vi "Straight Movement Simple.vi"() -> (3 "Finished?":bool)   [LabVIEW 2012]
uses:
  Robot Global Data.vi
  <vilib>/addons/control/pid/pid.llb/PID (DBL).vi
  <vilib>/addons/control/pid/NI_PID_pid.lvlib
panel:
  in  "Distance":dbl
  in  "Slow-down time":dbl
  in  "Speed-up time":dbl
  in  "Time":dbl
  in  "Spare Correction Time":dbl
  in  "Tolerance":dbl
  in  "Smooth Movment PID gains":T1={"proportional gain (Kc)"=1.0, "integral time (Ti, min)"=0.01, "derivative time (Td, min)"=0.0} {"derivative time (Td, min)" format="%.3f"; "integral time (Ti, min)" format="%.3f"; "proportional gain (Kc)" format="%.3f"}
  in  "Correction PID gains":T1={"proportional gain (Kc)"=1.0, "integral time (Ti, min)"=0.01, "derivative time (Td, min)"=0.0} {"derivative time (Td, min)" format="%.3f"; "integral time (Ti, min)" format="%.3f"; "proportional gain (Kc)" format="%.3f"}
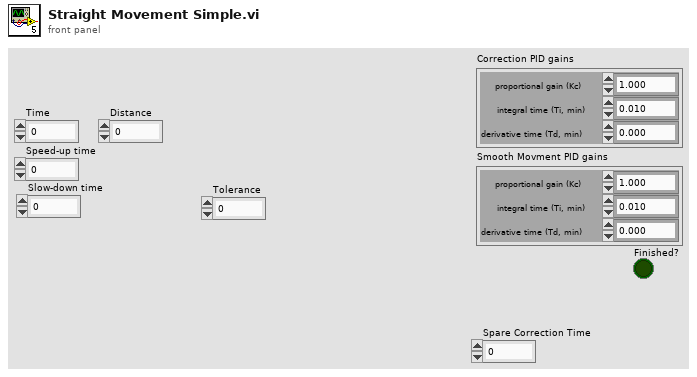
[diagram p1: front panel]
types:
  T1 = cluster{"proportional gain (Kc)":dbl, "integral time (Ti, min)":dbl, "derivative time (Td, min)":dbl}
  T2 = typedef "LoopDisable.ctl" = cluster{"Climb.vi":bool, "LauncherAngle.vi":bool, "Launcher.vi":bool, "ArmControl.vi":bool, "WinchMotor.vi":bool, "ReadDriveEncoder.vi":bool}
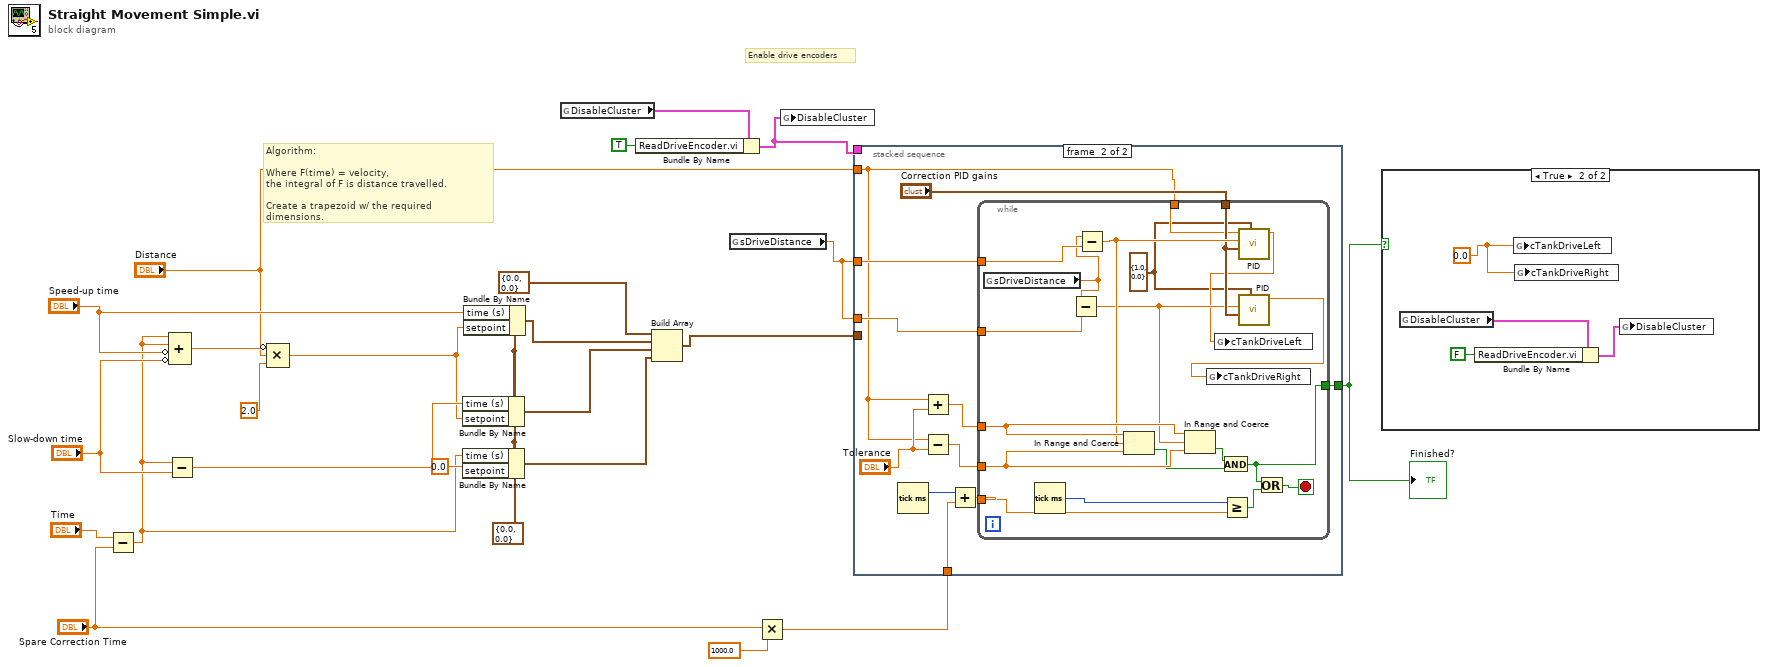
[diagram p0: block diagram]
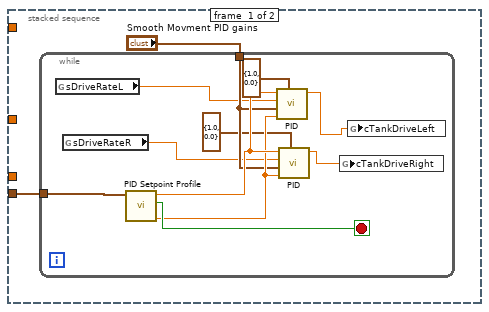
[diagram p3: hidden frame]
diagram:
  w10 = cluster{"time (s)":dbl, "setpoint":dbl} {"time (s)"=0.0, "setpoint"=0.0}
  # "Enable drive encoders"
  # "Algorithm:\n\nWhere F(time) = velocity,\nthe integral of F is distance travelled.\n\nCreate a trapezoid w/ the required dimensions."
  n1 = Subtract(x="Time", y="Spare Correction Time") -> (x-y=w12:dbl)
  n2 = Subtract(x=w12, y="Slow-down time") -> (x-y=w16:dbl)
  n3 = Compound Arithmetic op=ADD(w12, w12, invert "Speed-up time", invert "Slow-down time") -> (w8:dbl)
  n4 = Compound Arithmetic op=MULTIPLY(invert w8, "Distance", 2.0 ("value")) -> (w6:dbl)
  n5 = Bundle By Name(cluster=w10, "time (s)"=w16, "setpoint"=w6) -> (w11:cluster{"time (s)":dbl, "setpoint":dbl})
  n6 = Bundle By Name(cluster=w10, "time (s)"=w12, "setpoint"=0.0) -> (w18:cluster{"time (s)":dbl, "setpoint":dbl})
  n7 = Bundle By Name(cluster=w10, "time (s)"="Speed-up time", "setpoint"=w6) -> (w17:cluster{"time (s)":dbl, "setpoint":dbl})
  n8 = global read "Robot Global Data.vi" "DisableCluster"() -> (w3:T2)
  n9 = Bundle By Name(cluster=w3, "ReadDriveEncoder.vi"=TRUE) -> (w1:T2)
  n10 = Build Array(cluster{"time (s)":dbl, "setpoint":dbl} {"time (s)"=0.0, "setpoint"=0.0}, w17, w11, w18) -> (w20:cluster{"time (s)":dbl, "setpoint":dbl}[])
  n11 = global read "Robot Global Data.vi" "sDriveDistance"() -> (w4:dbl)
  n12 = Multiply(x="Spare Correction Time", y=1000.0) -> (x*y=w23:dbl)
  n13 = global write "Robot Global Data.vi" "DisableCluster"(w1) -> ()
  n14 = stacked-sequence {
    tunnel: w20 -> [w26 _]
    tunnel: w4 -> [_ w45]
    tunnel: w4 -> [_ w44]
    tunnel: w23 -> [_ w47]
    tunnel: [_ w42] -> w5
    tunnel: "Distance" -> [_ w38]
    tunnel: w1 -> [_ _]
    frame #0 {
      n15 = while {
        tunnel: w26 -> [w34]
        tunnel: "Smooth Movment PID gains" -> [w33]
        stop <- w37 stop-if-true
        n16 = global read "Robot Global Data.vi" "sDriveRateL"() -> (w27:dbl)
        n17 = global read "Robot Global Data.vi" "sDriveRateR"() -> (w28:dbl)
        n18 = call <vilib>:"PID Setpoint Profile.vi"("setpoint profile"=w34) -> ("dt out (s)"=w35:dbl, "profile complete?"=w37:bool, "setpoint"=w36:dbl)  [unwired: 5 in, 1 out]
        n19 = call-poly <vilib>:"PID.vi"("output range"=cluster{"output high":dbl, "output low":dbl} {"output high"=1.0, "output low"=0.0}, "dt (s)"=w35, "PID gains"=w33, "process variable"=w27, "setpoint"=w36) -> ("output"=w29:dbl)  [unwired: 5 in, 1 out]
        n20 = call-poly <vilib>:"PID.vi"("output range"=cluster{"output high":dbl, "output low":dbl} {"output high"=1.0, "output low"=0.0}, "dt (s)"=w35, "PID gains"=w33, "process variable"=w28, "setpoint"=w36) -> ("output"=w30:dbl)  [unwired: 5 in, 1 out]
        n21 = global write "Robot Global Data.vi" "cTankDriveRight"(w30) -> ()
        n22 = global write "Robot Global Data.vi" "cTankDriveLeft"(w29) -> ()
      }
    }
    frame #1 {
      n23 = Tick Count (ms)() -> (millisecond timer value=w48:u32)
      n24 = Add(x=w38, y="Tolerance") -> (x+y=w39:dbl)
      n25 = Subtract(x=w38, y="Tolerance") -> (x-y=w41:dbl)
      n26 = Add(x=w48, y=w47) -> (x+y=w46:dbl)
      n27 = while {
        tunnel: w46 -> [w64]
        tunnel: w45 -> [w63]
        tunnel: w44 -> [w55]
        tunnel: w39 -> [w61]
        tunnel: w41 -> [w62]
        tunnel: "Correction PID gains" -> [w57]
        tunnel: [w56] -> w42
        tunnel: w38 -> [w53]
        stop <- w67 stop-if-true
        w49 = cluster{"output high":dbl, "output low":dbl} {"output high"=1.0, "output low"=0.0} ("output range")
        n28 = global read "Robot Global Data.vi" "sDriveDistance"() -> (w52:dbl)
        n29 = Tick Count (ms)() -> (millisecond timer value=w65:u32)
        n30 = Subtract(x=w52, y=w55) -> (x-y=w54:dbl)
        n31 = Subtract(x=w52, y=w63) -> (x-y=w60:dbl)
        n32 = In Range and Coerce(upper limit=w61, x=w60, lower limit=w62) -> (In Range?=w59:bool)  [unwired: 1 out]
        n33 = In Range and Coerce(upper limit=w61, x=w54, lower limit=w62) -> (In Range?=w58:bool)  [unwired: 1 out]
        n34 = And(x=w58, y=w59) -> (x .and. y?=w56:bool)
        n35 = Greater Or Equal?(x=w65, y=w64) -> (x >= y?=w66:bool)
        n36 = call-poly <vilib>:"PID.vi"("output range"=w49, "PID gains"=w57, "process variable"=w60, "setpoint"=w53) -> ("output"=w51:dbl)  [unwired: 6 in, 1 out]
        n37 = global write "Robot Global Data.vi" "cTankDriveLeft"(w51) -> ()
        n38 = call-poly <vilib>:"PID.vi"("output range"=w49, "PID gains"=w57, "process variable"=w54) -> ("output"=w50:dbl)  [unwired: 7 in, 1 out]
        n39 = global write "Robot Global Data.vi" "cTankDriveRight"(w50) -> ()
        n40 = Or(x=w56, y=w66) -> (x .or. y?=w67:bool)
      }
    }
  }
  "Finished?" <- w5
  n41 = case shown="True" w5 {
    frame False {
    }
    frame True {
      w71 = 0.0 ("Left axis value")
      n42 = global read "Robot Global Data.vi" "DisableCluster"() -> (w70:T2)
      n43 = Bundle By Name(cluster=w70, "ReadDriveEncoder.vi"=FALSE) -> (w69:T2)
      n44 = global write "Robot Global Data.vi" "cTankDriveLeft"(w71) -> ()
      n45 = global write "Robot Global Data.vi" "cTankDriveRight"(w71) -> ()
      n46 = global write "Robot Global Data.vi" "DisableCluster"(w69) -> ()
    }
  }
